vi "Dé électronique .vi"() -> ()   [LabVIEW 2018]
panel:
  out "Boolean":bool
  in  "Chiffre":ext
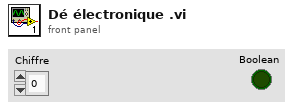
[diagram p1: front panel]
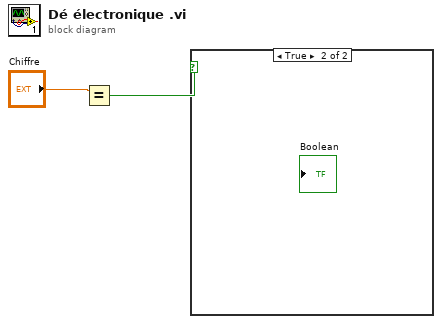
[diagram p0: block diagram]
diagram:
  n1 = Equal?(x="Chiffre") -> (x = y?=w1:bool)  [unwired: 1 in]
  n2 = case shown="True" w1 {
    frame False {
    }
    frame True {
    }
  }
